vi "Phantom v7.3 lightweight controller.vi"() -> ()   [LabVIEW 2014]
uses:
  Program Files (x86)/National Instruments/LabVIEW 2011/instr.lib/Vision Research Phantom Series Labview Driver/_Type Defs/PHCon ACQUIPARAMS.ctl
  Program Files (x86)/National Instruments/LabVIEW 2011/instr.lib/Vision Research Phantom Series Labview Driver/_Type Defs/PhCon SyncImaging.ctl
  Program Files (x86)/National Instruments/LabVIEW 2011/instr.lib/Vision Research Phantom Series Labview Driver/_Type Defs/Rect.ctl
  Program Files (x86)/National Instruments/LabVIEW 2011/instr.lib/Vision Research Phantom Series Labview Driver/_Type Defs/PHCon Time64.ctl
  Program Files (x86)/National Instruments/LabVIEW 2011/instr.lib/Vision Research Phantom Series Labview Driver/_Type Defs/PhInt CFA.ctl
  Program Files (x86)/National Instruments/LabVIEW 2011/instr.lib/Vision Research Phantom Series Labview Driver/_Type Defs/enum buttons.ctl
  Program Files (x86)/National Instruments/LabVIEW 2011/instr.lib/Vision Research Phantom Series Labview Driver/_Type Defs/Point.ctl
  Program Files (x86)/National Instruments/LabVIEW 2011/instr.lib/Vision Research Phantom Series Labview Driver/_Type Defs/StampTime.ctl
  Program Files (x86)/National Instruments/LabVIEW 2011/instr.lib/Vision Research Phantom Series Labview Driver/_Type Defs/PHCon CINESTATUS.ctl
  Program Files (x86)/National Instruments/LabVIEW 2011/instr.lib/Vision Research Phantom Series Labview Driver/_Type Defs/PhCon Predefined Cines.ctl
  Program Files (x86)/National Instruments/LabVIEW 2011/instr.lib/Vision Research Phantom Series Labview Driver/_Type Defs/PHCon IMRANGE.ctl
  Program Files (x86)/National Instruments/LabVIEW 2011/instr.lib/Vision Research Phantom Series Labview Driver/_Type Defs/PhFile InfName.ctl
  Program Files (x86)/National Instruments/LabVIEW 2011/instr.lib/Vision Research Phantom Series Labview Driver/_Type Defs/PhInt PhProcessImage Selectors.ctl
panel:
  in  "Use timer":bool=TRUE
  out "Datarun timed out":bool
  in  "Save interval (shots)":u32
  out "Data run info":T1
  out "Run datasocket error":errorcluster
  in  "Zoom Factor":sgl(slide)=1.0 scale=0.0..10.0
  in  "Start recording":bool
  out "Last recording time":timestamp
  in  "Seconds between recordings":dbl format="%#_13g"
  out "Save path":path
  in  "Take picture":bool
  out "state":T2(ring)
  in  "Black Ref":bool
  in  "Recording":bool caption="Record?"
  out "Cine 1 Status":T3
  in  "Number of shots":i32
  in  "Frames After \nTrigger":i32
  in  "Frames Before \nTrigger":i32
  in  "Save StampTime":T4
  out "Save Progress":u8(slide) max=100 scale=0.0..100.0
  out "Error":errorcluster
  in  "error in":errorcluster
  out "Continue":bool
  in  "EXIT":bool
  in  "Trigger":bool
  in  "Update":bool
  in  "Parameters":T5
  out "Preview":picture
  out "CAR":T6[](array[typedef])
  in  "Current State":T7
  out "Serial":u32
  out "Camera Name":string
  out "Parameters":T8 {"CFA"."CFA" items=["CFA_NONE", "CFA_VRI", "CFA_VRIV6", "CFA_BAYER", "CFA_BAYERFLIP"]; "TriggerTime"."fractions" format="%32.0f"}
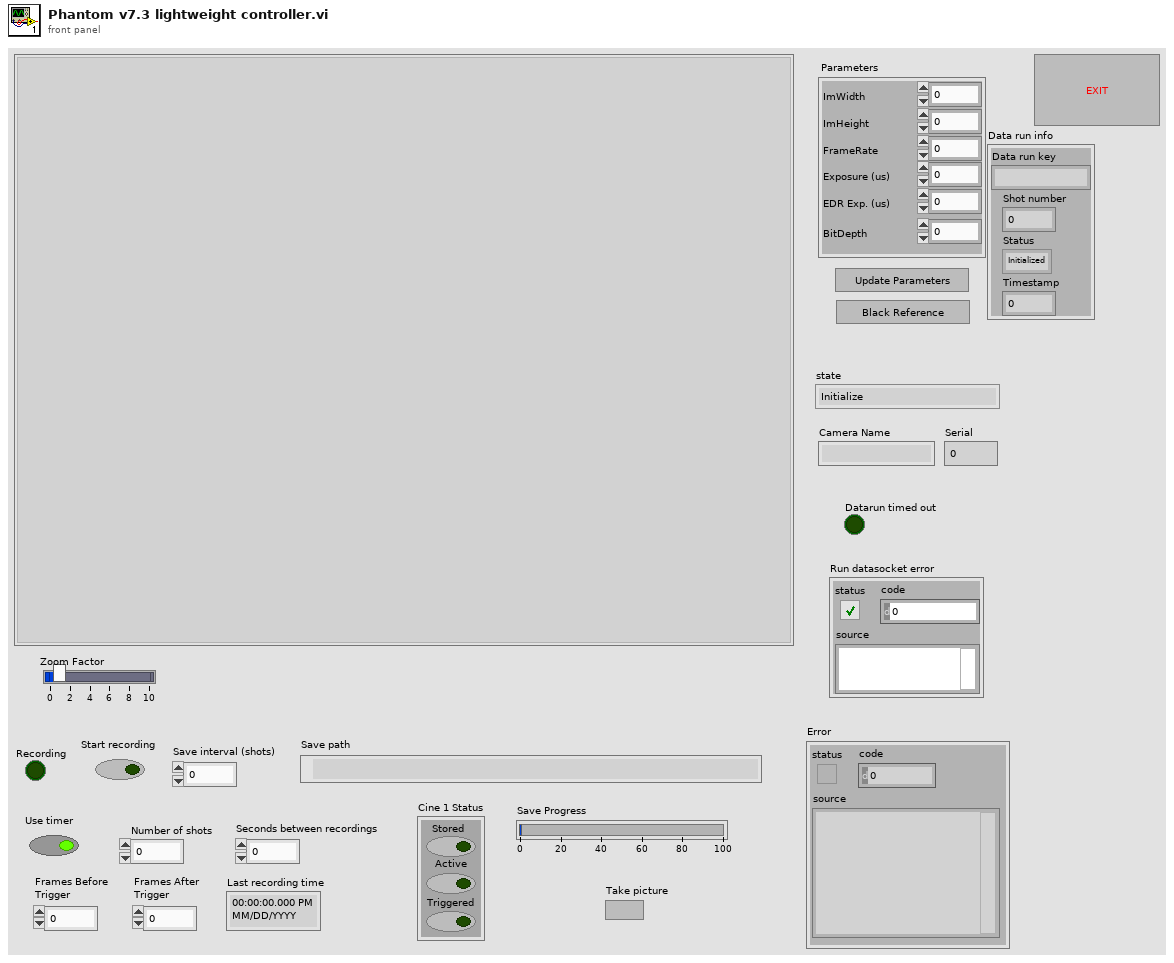
[diagram p1: front panel]
types:
  T1 = cluster{"Data run key":string, "Shot number":u32, "Status":enum16{"Initialized", "Running", "Aborted", "Default"}, "Timestamp":dbl}
  T2 = enum16{"Initialize", "Wait for Action", "Update", "Black Ref", "CTS", "Review", "End"}
  T3 = typedef "PHCon CINESTATUS.ctl" = cluster{"Stored":bool, "Active":bool, "Triggered":bool}
  T4 = typedef "StampTime.ctl" = enum32{"NoTimeStamp", "Time stamp", "", "Time stamp from trigger"}
  T5 = cluster{"ImWidth":u32, "ImHeight":u32, "FrameRate":u32, "Exposure (us)":u32, "EDR Exp. (us)":u32, "BitDepth":u32}
  T6 = typedef "Point.ctl" = cluster{"X":i32, "Y":i32}
  T7 = typedef "enum buttons.ctl" = enum16{"Initialize", "Wait for Action", "Update", "Capture", "Trigger", "Open Cine", "Save Cine", "CTS", "End"}
  T8 = typedef "PHCon ACQUIPARAMS.ctl" = cluster{"ImWidth":u32, "ImHeight":u32, "FrameRate":u32, "Exposure":u32, "EDRExposure":u32, "ImDelay":u32, "PTFrames":u32, "ImCount":u32, "SyncImaging":T9, "AutoExposure":u32, "AutoExpLevel":u32, "AutoExpSpeed":u32, "AutoExpRect":T10, "Recorded":bool, "TriggerTime":T11, "RecordedCount":u32, "FirstIm":i32, "FRPSteps":u32, "FRPImgNr":i32[], "FRPRate":u32[], "FRPExp":u32[], "Decimation":u32, "BitDepth":u32, "CamGainRed":u32, "CamGainGreen":u32, "CamGainBlue":u32, "CamGain":u32, "ShutterOff":bool, "CFA":T12, "CineName[256]":u8[], "Description[4096]":u8[], "FRPShape [16]":u32[]}
  T9 = typedef "PhCon SyncImaging.ctl" = enum32{"SYNC_INTERNAL", "SYNC_EXTERNAL", "SYNC_LOCKTOIRIG"}
  T10 = typedef "Rect.ctl" = cluster{"X":i32, "Y":i32, "Width":i32, "Height":i32}
  T11 = typedef "PHCon Time64.ctl" = cluster{"fractions":u32, "seconds":u32}
  T12 = typedef "PhInt CFA.ctl" = cluster{"CFA":u32, "VRIV6 Mask":cluster{"TL_GRAY":bool, "TR_GRAY":bool, "BL_GRAY":bool, "BR_GRAY":bool}}
  T13 = enum16{"Initialized", "Running", "Aborted", "Default"}
  T14 = cluster{"ImWidth":u32, "ImHeight":u32, "FrameRate":u32, "Exposure (us)":u32, "EDR Exp. (us)":u32, "ImDelay":u32, "Post Trig. Frames":u32, "ImCount":u32, "BitDepth":u32}
  T15 = typedef "PhCon Predefined Cines.ctl" = i32
  T16 = cluster{"pCS[0]":T3, "pCS[1]":T3, "pCS[2]":T3, "pCS[3]":T3, "pCS[4]":T3, "pCS[5]":T3, "pCS[6]":T3, "pCS[7]":T3, "pCS[8]":T3}
  T17 = typedef "PhInt PhProcessImage Selectors.ctl" = u16
  T18 = typedef "PhFile InfName.ctl" = u32
  T19 = typedef "PHCon IMRANGE.ctl" = cluster{"First":i32, "Cnt":u32}
  T20 = typedef "BITMAPINFO.ctl" = cluster{"BITMAPINFOHEADER":T21, "RGB Map":T22[]}
  T21 = typedef "BITMAPINFOHEADER.ctl" = cluster{"biSize":u32, "biWidth":i32, "biHeight":i32, "biPlanes":u16, "biBitCount":u16, "biCompression":u32, "biSizeImage":u32, "biXPelsPerMeter":i32, "biYPelsPerMeter":i32, "biClrUsed":u32, "biClrImportant":u32}
  T22 = typedef "RGBQUAD.ctl" = cluster{"rgbBlue":u8, "rgbGreen":u8, "rgbRed":u8, "rgbResevered":u8}
  T23 = typedef "PhInt IH.ctl" = cluster{"biSize":u32, "biWidth":i32, "biHeight":i32, "biPlanes":u16, "biBitCount":u16, "biCompresssion":u32, "biSizeImage":u32, "biXPelsPerMeter":i32, "biYPelsPerMeter":i32, "biClrUsed":u32, "biClrImportant":u32, "BlackLevel":i32, "WhiteLevel":i32}
  T24 = typedef "PHCon CAMERAOPTIONS.ctl" = cluster{"OSD":u32, "VideoSystem":T25, "ModulatedIRIG":bool, "RisingEdge":bool, "FilterTime":u32, "MemGate":bool, "StartInRec":bool, "Color":bool, "TestImage":bool, "OSDColor [8]":T22[], "OSDOpaque":bool, "OSDLeft":i32, "OSDTop":i32, "OSDBottom":i32, "ImageX":i32, "ImageY":i32, "AutoSaveNVM":bool, "AutoSaveFile":bool, "AutoPlay":bool, "AutoCapture":bool, "Filename":u8[], "SaveRng":T19, "LongReady":bool, "RealTimeOutput":bool, "RangeData":u32, "SourceCamSer":u32, "SliceNr":u32, "SliceCnt":u32, "FRPi3Trig":bool, "UT":u32, "AutoSaveFormat":i8, "SourceCamVer":u32, "RAMBitDepth":u32, "VideoTone":i32, "VideoZoom":i32, "FormatWidth":i32, "FormatHeight":i32, "AutoPlayCnt":u32, "OSDDisable":u32, "RecToMag":bool, "IrigOut":bool, "FormatXOffset":i32, "FormatYOffset":i32}
  T25 = typedef "PhCon VideoSystem.ctl" = u32
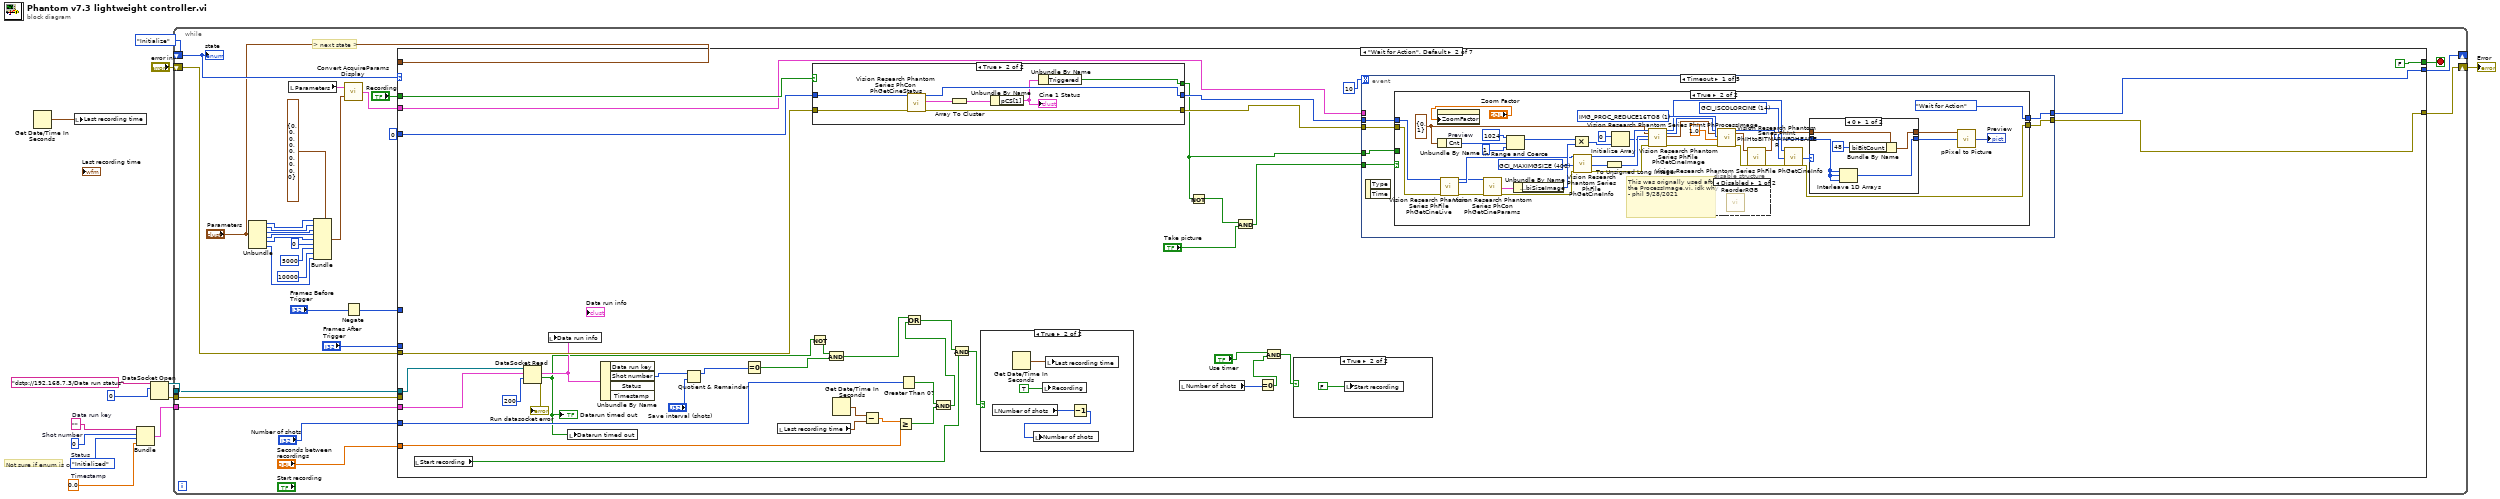
[diagram p0: block diagram]
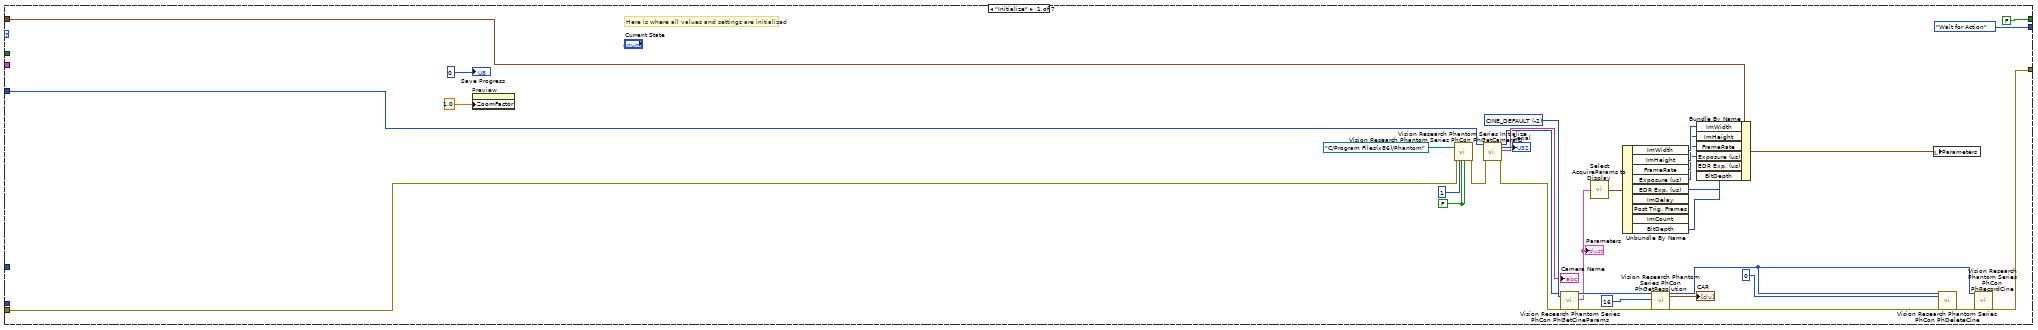
[diagram p2: hidden frame]
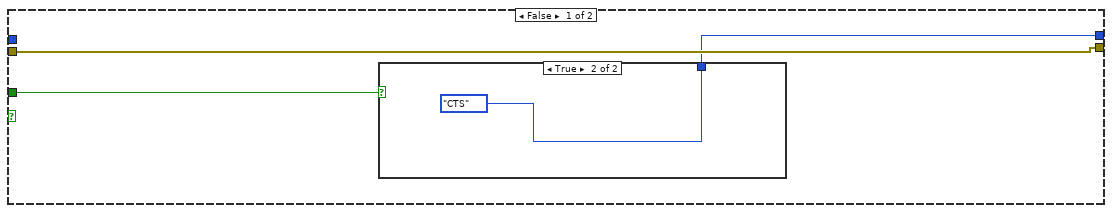
[diagram p5: hidden frame]
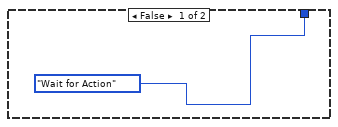
[diagram p6: hidden frame]
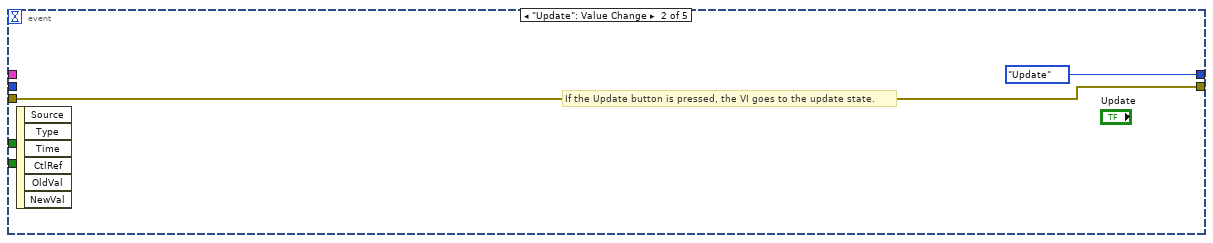
[diagram p9: hidden frame]
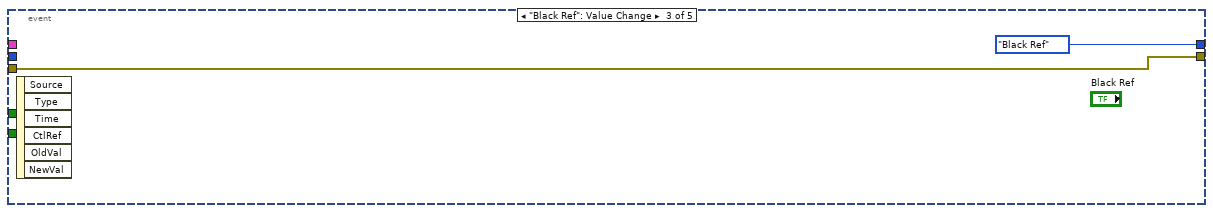
[diagram p10: hidden frame]
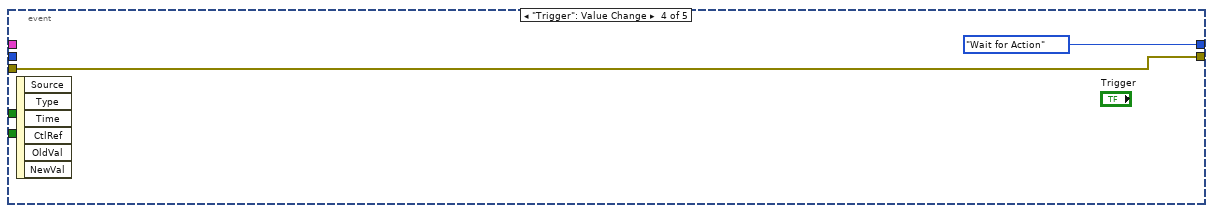
[diagram p11: hidden frame]
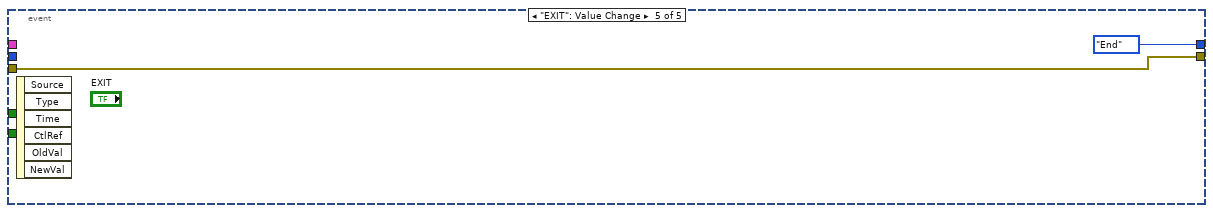
[diagram p12: hidden frame]
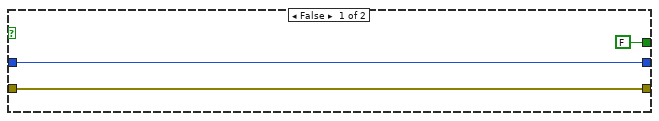
[diagram p13: hidden frame]
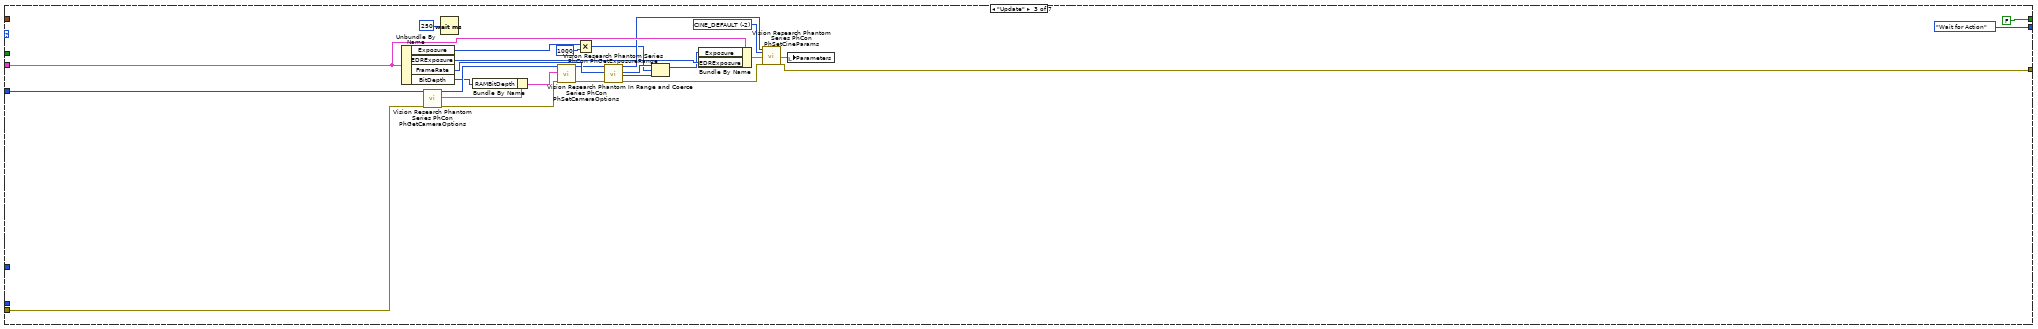
[diagram p14: hidden frame]
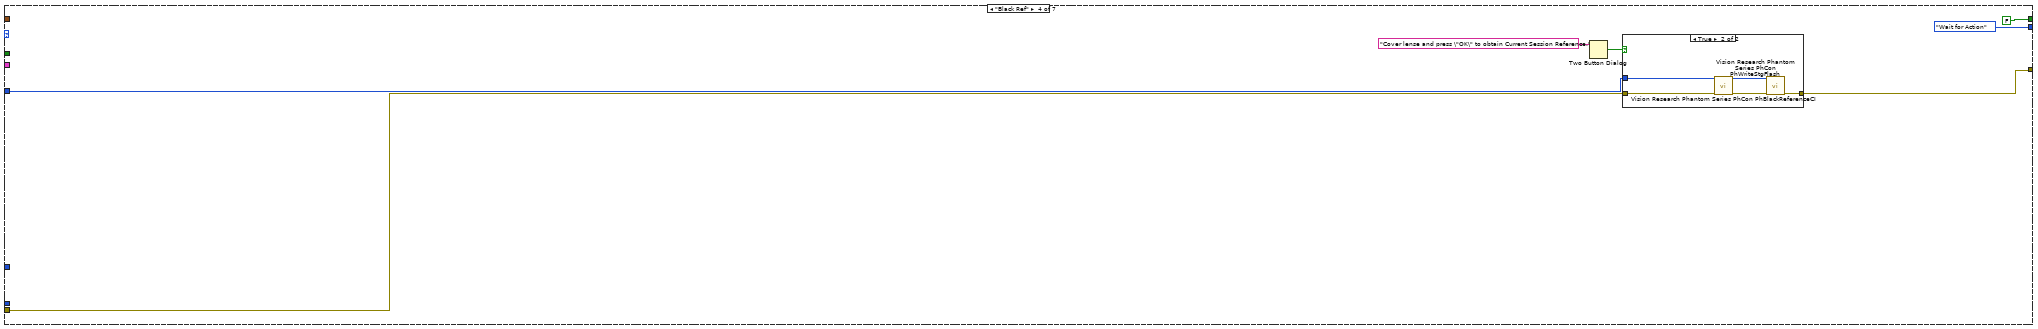
[diagram p15: hidden frame]
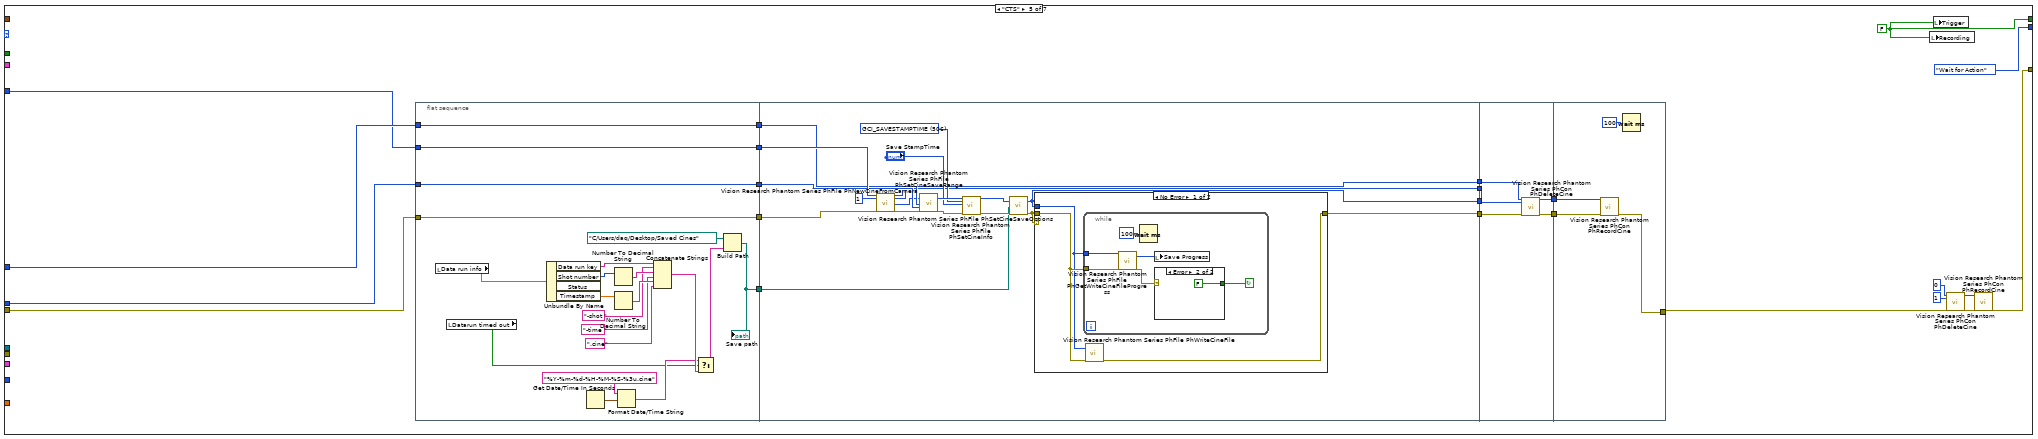
[diagram p17: hidden frame]
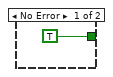
[diagram p18: hidden frame]
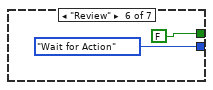
[diagram p20: hidden frame]
diagram:
  w8 = 0.0  # Timestamp
  w7 = T13."Initialized"  # Status
  w6 = u32 0  # Shot number
  w5 = ""  # Data run key
  # "Not sure if enum is correct"
  n1 = Get Date/Time In Seconds() -> (seconds since 1Jan1904=w1:timestamp)
  n2 = local write "Last recording time"(w1) -> ()
  n3 = Bundle("Data run key"=w5, "Shot number"=w6, "Status"=w7, "Timestamp"=w8) -> (w4:T1)  [unwired: 1 in]
  n4 = DataSocket Open(10:0, 11:"dstp://192.168.7.3/Data run status") -> (0:w2:errorcluster, 3:w3:refnum<k13>)  [unwired: 2 in]
  n5 = while {
    shift-right: [w42] -> _
    shift-left: T2."Initialize" -> [w41]
    shift-right: [w39] -> w13
    shift-left: "error in" -> [w31]
    tunnel: w3 -> [w18]
    tunnel: w4 -> [w17]
    tunnel: w2 -> [w16]
    stop <- w40 stop-if-true
    # "> next state >"
    n6 = Unbundle("Parameters") -> ("ImWidth"=w30:u32, "ImHeight"=w29:u32, "FrameRate"=w28:u32, "Exposure (us)"=w27:u32, "EDR Exp. (us)"=w26:u32, "BitDepth"=w21:u32)
    n7 = local read "Parameters"() -> (w37:T8)
    n8 = Bundle(cluster=T14 {"ImWidth"=0, "ImHeight"=0, "FrameRate"=0, "Exposure (us)"=0, "EDR Exp. (us)"=0, "ImDelay"=0, "Post Trig. Frames"=0, "ImCount"=0, "BitDepth"=0} ("ACQUIPARAMS Display"), "ImWidth"=w30, "ImHeight"=w29, "FrameRate"=w28, "Exposure (us)"=w27, "EDR Exp. (us)"=w26, "ImDelay"=u32 0 ("x"), "Post Trig. Frames"=u32 5000 ("x"), "ImCount"=u32 10000 ("x"), "BitDepth"=w21) -> (w22:T14)
    n9 = call "Convert AcquireParams Display.vi"("ACQUIPARAMS Display"=w22, "ACQUIPARAMS [in]"=w37) -> ("ACQUIPARAMS [out]"=w38:T8)
    n10 = Negate(x="Frames Before \nTrigger") -> (-x=w32:i32)
    n11 = case shown="\"Wait for Action\", Default" w41 {
      selector: w41 -> [_ _ _ _ _ _ w331]
      tunnel: w38 -> [_ w109 w223 _ _ _ _]
      tunnel: [T2."Wait for Action" w105 T2."Wait for Action" T2."Wait for Action" T2."Wait for Action" T2."Wait for Action" w331] -> w42
      tunnel: [FALSE FALSE FALSE FALSE w256 FALSE TRUE] -> w40
      tunnel: w31 -> [w61 w117 w208 w230 w249 _ w329]
      tunnel: [w58 w106 w221 w229 w262 _ w327] -> w39
      tunnel: u32 0 ("Camera Number") -> [w66 w116 w207 w231 w246 _ _]
      tunnel: "Frames After \nTrigger" -> [_ _ _ _ w247 _ _]
      tunnel: w32 -> [_ _ _ _ w248 _ _]
      tunnel: "Recording" -> [_ w115 _ _ _ _ _]
      tunnel: "Parameters" -> [w44 _ _ _ _ _ _]
      tunnel: w18 -> [_ w93 _ _ _ _ _]
      tunnel: w17 -> [_ w92 _ _ _ _ _]
      tunnel: w16 -> [_ _ _ _ _ _ _]
      tunnel: "Number of shots" -> [_ w103 _ _ _ _ _]
      tunnel: "Seconds between recordings" -> [_ w99 _ _ _ _ _]
      frame "Initialize" {
        w69 = FALSE ("ID Query (T: Check)")
        w72 = T15 -2 items=["CINE_DEFAULT "=-2, "CINE_CURRENT "=-1, "CINE_PREVIEW  "=0, "CINE_FIRST    "=1] ("Cine")
        # "Here is where all values and settings are initialized"
        n12 = property on="Preview" class="Pict"("ZoomFactor"=sgl 1.0 ("Zoom Factor")) -> ()  [unwired: 2 in, 2 out]
        n13 = call "Vision Research Phantom Series Initialize.vi"("Storage Path (\"\")"=path "C:/Program Files(x86)/Phantom" ("Storage Path (\"\")"), "error in (no error)"=w61, "CallID"=u32 1, "ID Query (T: Check)"=w69, "Reset (F: Don't Reset)"=w69) -> ("Error Out"=w68:errorcluster)  [unwired: 14 out]
        n14 = call "Vision Research Phantom Series PhCon PhGetCameraID.vi"("CN in"=w66, "Error In (no error)"=w68) -> ("CN out"=w59:u32, "pSerial"=→"Serial":u32, "pCameraName"=→"Camera Name":string, "Error Out"=w60:errorcluster)  [unwired: 1 in, 13 out]
        n15 = call "Vision Research Phantom Series PhCon PhGetCineParams.vi"("CN in"=w59, "Cine"=w72, "Error In (no error)"=w60) -> ("CN out"=w75:u32, "ACQUIPARAMS"=w64:T8, "Error Out"=w65:errorcluster)  [unwired: 1 in, 13 out]
        "Parameters" <- w64
        n16 = call "Select AcquireParams to Display.vi"("ACQUIPARAMS"=w64) -> ("ACQUIPARAMS Display"=w51:T14)
        n17 = Unbundle By Name(w51) -> ("ImWidth"=w50:u32, "ImHeight"=w49:u32, "FrameRate"=w48:u32, "Exposure (us)"=w47:u32, "EDR Exp. (us)"=w45:u32, "BitDepth"=w46:u32)  [unwired: 3 out]
        n18 = call "Vision Research Phantom Series PhCon PhGetResolution.vi"("CN in"=w75, "pCnt"=16, "Error In (no error)"=w65) -> ("CN out"=w56:u32, "CAR"=→"CAR":T6[], "Error Out"=w55:errorcluster)  [unwired: 2 in, 12 out]
        n19 = Bundle By Name(cluster=w44, "ImWidth"=w50, "ImHeight"=w49, "FrameRate"=w48, "Exposure (us)"=w47, "EDR Exp. (us)"=w45, "BitDepth"=w46) -> (w43:T5)
        n20 = local write "Parameters"(w43) -> ()
        n21 = call "Vision Research Phantom Series PhCon PhDeleteCine.vi"("CN in"=w56, "Cine"=0, "Error In (no error)"=w55) -> ("Error Out"=w54:errorcluster)  [unwired: 15 in, 1 out]
        n22 = call "Vision Research Phantom Series PhCon PhRecordCine.vi"("CN in"=w56, "Error In (no error)"=w54) -> ("Error Out"=w58:errorcluster)  [unwired: 1 in, 16 out]
        "Save Progress" <- u8 0 ("Value")
      }
      frame "Wait for Action", Default {
        n23 = local read "Start recording"() -> (w81:bool)
        n24 = DataSocket Read(9:200, 10:w92, 11:w93) -> (0:→"Run datasocket error":errorcluster, 1:w86:bool, 2:w91:T1)  [unwired: 2 in, 4 out]
        "Datarun timed out" <- w86
        n25 = local write "Data run info"(w91) -> ()
        n26 = local write "Datarun timed out"(w86) -> ()
        n27 = Unbundle By Name(w91) -> ("Shot number"=w90:u32)  [unwired: 3 out]
        n28 = Quotient & Remainder(x=w90, y="Save interval (shots)") -> (x-y*floor(x/y)=w88:u32)  [unwired: 1 out]
        n29 = Equal To 0?(x=w88) -> (x = 0?=w87:bool)
        n30 = local read "Last recording time"() -> (w101:timestamp)
        n31 = Not(x=w86) -> (.not. x?=w85:bool)
        n32 = case shown="True" w115 {
          tunnel: w117 -> [w191 w199]
          tunnel: w116 -> [w190 w198]
          tunnel: [w190 w197] -> w108
          tunnel: [FALSE ("Triggered") w193] -> w104
          tunnel: [w191 w192] -> w107
          frame False {
          }
          frame True {
            n33 = call "Vision Research Phantom Series PhCon PhGetCineStatus.vi"("CN in"=w198, "Error In (no error)"=w199) -> ("CN out"=w197:u32, "pCS"=w196:T3[], "Error Out"=w192:errorcluster)  [unwired: 15 in]
            n34 = Array To Cluster(array=w196) -> (cluster=w195:T16)
            n35 = Unbundle By Name(w195) -> ("pCS[1]"=w194:T3)
            "Cine 1 Status" <- w194
            n36 = Unbundle By Name(w194) -> ("Triggered"=w193:bool)
          }
        }
        n37 = And(x=w85, y=w87) -> (x .and. y?=w84:bool)
        n38 = Get Date/Time In Seconds() -> (seconds since 1Jan1904=w102:timestamp)
        n39 = Subtract(x=w102, y=w101) -> (x-y=w100:dbl)
        n40 = Greater Or Equal?(x=w100, y=w99) -> (x >= y?=w97:bool)
        n41 = Greater Than 0?(x=w103) -> (x > 0?=w98:bool)
        n42 = And(x=w98, y=w97) -> (x .and. y?=w83:bool)
        n43 = Or(x=w84, y=w83) -> (x .or. y?=w82:bool)
        n44 = And(x=w82, y=w81) -> (x .and. y?=w80:bool)
        n45 = case shown="True" w80 {
          frame False {
          }
          frame True {
            n46 = local read "Number of shots"() -> (w121:i32)
            n47 = Get Date/Time In Seconds() -> (seconds since 1Jan1904=w120:timestamp)
            n48 = local write "Recording"(TRUE ("Record?")) -> ()
            n49 = local write "Last recording time"(w120) -> ()
            n50 = Decrement(x=w121) -> (x-1=w119:i32)
            n51 = local write "Number of shots"(w119) -> ()
          }
        }
        n52 = local read "Number of shots"() -> (w96:i32)
        n53 = Not(x=w104) -> (.not. x?=w112:bool)
        n54 = And(x=w112, y="Take picture") -> (x .and. y?=w110:bool)
        n55 = Equal To 0?(x=w96) -> (x = 0?=w78:bool)
        n56 = And(x="Use timer", y=w78) -> (x .and. y?=w77:bool)
        n57 = case shown="True" w77 {
          frame False {
          }
          frame True {
            n58 = local write "Start recording"(FALSE ("Start recording")) -> ()
          }
        }
        n59 = event shown="[0] Timeout" {
          selector: _ -> [_ _ _ _ _]
          dyn-events: _ -> [_ _ _ _ _]
          timeout: 10 -> [_ _ _ _ _]
          tunnel: [w125 T2."Update" T2."Black Ref" T2."Wait for Action" T2."End"] -> w105
          tunnel: w107 -> [w127 w182 w183 w186 w188]
          tunnel: [w128 w182 w183 w186 w188] -> w106
          tunnel: w109 -> [_ _ _ _ _]
          tunnel: w108 -> [w126 _ _ _ _]
          tunnel: w110 -> [w124 _ _ _ _]
          tunnel: w104 -> [w123 _ _ _ _]
          event Timeout {
            n60 = event-data() -> ()  [unwired: 3 out]
            n61 = case shown="True" w124 {
              tunnel: [w131 w153] -> w128
              tunnel: w127 -> [w131 w149]
              tunnel: w126 -> [_ w148]
              tunnel: [w129 T2."Wait for Action"] -> w125
              tunnel: w123 -> [w130 _]
              frame False {
                n62 = case shown="True" w130 {
                  tunnel: [T2."Wait for Action" T2."CTS"] -> w129
                  frame False {
                  }
                  frame True {
                  }
                }
              }
              frame True {
                w155 = T17 1 items=["IMG_PROC_REDUCE16TO8"=1] ("procID")
                w158 = T18 14 items=["GCI_CFA"=0, "GCI_FRAMERATE"=1, "GCI_EXPOSURE"=2, "GCI_AUTOEXPOSURE"=3, "GCI_REALBPP"=4, "GCI_CAMERASERIAL"=5, "GCI_HEADSERIAL0"=6, "GCI_HEADSERIAL1"=7, "GCI_HEADSERIAL2"=8, "GCI_HEADSERIAL3"=9, "GCI_TRIGTIMESEC"=10, "GCI_TRIGTIMEFR"=11, "GCI_ISFILECINE"=12, "GCI_IS16BPPCINE"=13, "GCI_ISCOLORCINE"=14, "GCI_ISMULTIHEADCINE"=15, "GCI_EXPOSURENS"=16, "GCI_EDREXPOSURENS"=17, "GCI_FRAMEDELAYNS"=19, "GCI_FROMFILETYPE"=20, "GCI_COMPRESSION"=21, "GCI_CAMERAVERSION"=22, "GCI_ROTATE"=23, "GCI_IMWIDTH"=24, "GCI_IMHEIGHT"=25, "GCI_IMWIDTHACQ"=26, "GCI_IMHEIGHTACQ"=27, "GCI_POSTTRIGGER"=28, "GCI_IMAGECOUNT"=29, "GCI_TOTALIMAGECOUNT"=30, "GCI_TRIGFRAME"=31, "GCI_AUTOEXPLEVEL"=32, "GCI_AUTOEXPTOP"=33, "GCI_AUTOEXPLEFT"=34, "GCI_AUTOEXPBOTTOM"=35, "GCI_AUTOEXPRIGHT"=36, "GCI_RECORDINGTIMEZONE"=37, "GCI_FIRSTIMAGENO"=38, "GCI_FIRSTMOVIEIMAGE"=39, "GCI_CINENAME"=40, "GCI_FRPSTEPS"=100, "GCI_FRP1X"=101, "GCI_FRP1Y"=102, "GCI_FRP2X"=103, "GCI_FRP2Y"=104, "GCI_FRP3X"=105, "GCI_FRP3Y"=106, "GCI_FRP4X"=107, "GCI_FRP4Y"=108, "GCI_WRITEERR"=109, "GCI_LENSDESCRIPTION"=110, "GCI_LENSAPERATURE"=111, "GCI_LENSFOCALLENGTH"=112, "GCI_WB"=200, "GCI_WBVIEW"=201, "GCI_BRIGHT"=202, "GCI_CONTRAST"=203, "GCI_GAMMA"=204, "GCI_GAMMAR"=223, "GCI_GAMMAB"=224, "GCI_SATURATION"=205, "GCI_HUE"=206, "GCI_FLIPH"=207, "GCI_FLIPV"=208, "GCI_FILTERCODE"=209, "GCI_IMFILTER"=210, "GCI_INTALGO"=211, "GCI_PEDESTALR"=212, "GCI_PEDESTALG"=213, "GCI_PEDESTALB"=214, "GCI_FLARE"=225, "GCI_CHROMA"=226, "GCI_TONE"=227, "GCI_ENABLEMATRICES"=228, "GCI_USERMATRIX"=229, "GCI_RESAMPLEACTIVE"=215, "GCI_RESAMPLEWIDTH"=216, "GCI_RESAMPLEHEIGHT"=217, "GCI_CROPACTIVE"=218, "GCI_CROPRECTANGLE"=219, "GCI_OFFSET16_8"=220, "GCI_GAIN16_8"=221, "GCI_DEMOSAICINGFUNCPTR"=222, "GCI_VFLIPVIEWACTIVE"=300, "GCI_MAXIMGSIZE"=400, "GCI_FRPIMGNOARRAY"=450, "GCI_FRPRATEARRAY"=451, "GCI_FRPSHAPEARRAY"=452, "GCI_TRIGTC"=470, "GCI_TRIGTCU"=471, "GCI_PBRATE"=472, "GCI_TCRATE"=473, "GCI_SAVERANGE"=500, "GCI_SAVEFILENAME"=501, "GCI_SAVEFILETYPE"=502, "GCI_SAVE16BIT"=503, "GCI_SAVEPACKED"=504, "GCI_SAVEXML"=505, "GCI_SAVESTAMPTIME"=506, "GCI_SAVEAVIFRAMERATE"=520, "GCI_SAVEAVICOMPRESSORLIST"=521, "GCI_SAVEAVICOMPRESSORINDEX"=522, "GCI_SAVEDPXLSB"=530, "GCI_SAVEDPXTO10BPS"=531, "GCI_SAVEDPXDATAPACKING"=532, "GCI_SAVEDPX10BITLOG"=533, "GCI_SAVEDPXEXPORTLOGLUT"=534, "GCI_SAVEDPX10BITLOGREFWHITE"=535, "GCI_SAVEDPX10BITLOGREFBLACK"=536, "GCI_SAVEDPX10BITLOGGAMMA"=537, "GCI_SAVEDPX10BITLOGFILMGAMMA"=538, "GCI_SAVEQTPLAYBACKRATE"=550, "GCI_SAVECCIQUALITY"=560, "GCI_UNCALIBRATEDIMAGE"=600, "GCI_NOPROCESSING"=601, "GCI_BADPIXELREPAIR"=602] ("InfName")
                w173 = T18 400 items=["GCI_CFA"=0, "GCI_FRAMERATE"=1, "GCI_EXPOSURE"=2, "GCI_AUTOEXPOSURE"=3, "GCI_REALBPP"=4, "GCI_CAMERASERIAL"=5, "GCI_HEADSERIAL0"=6, "GCI_HEADSERIAL1"=7, "GCI_HEADSERIAL2"=8, "GCI_HEADSERIAL3"=9, "GCI_TRIGTIMESEC"=10, "GCI_TRIGTIMEFR"=11, "GCI_ISFILECINE"=12, "GCI_IS16BPPCINE"=13, "GCI_ISCOLORCINE"=14, "GCI_ISMULTIHEADCINE"=15, "GCI_EXPOSURENS"=16, "GCI_EDREXPOSURENS"=17, "GCI_FRAMEDELAYNS"=19, "GCI_FROMFILETYPE"=20, "GCI_COMPRESSION"=21, "GCI_CAMERAVERSION"=22, "GCI_ROTATE"=23, "GCI_IMWIDTH"=24, "GCI_IMHEIGHT"=25, "GCI_IMWIDTHACQ"=26, "GCI_IMHEIGHTACQ"=27, "GCI_POSTTRIGGER"=28, "GCI_IMAGECOUNT"=29, "GCI_TOTALIMAGECOUNT"=30, "GCI_TRIGFRAME"=31, "GCI_AUTOEXPLEVEL"=32, "GCI_AUTOEXPTOP"=33, "GCI_AUTOEXPLEFT"=34, "GCI_AUTOEXPBOTTOM"=35, "GCI_AUTOEXPRIGHT"=36, "GCI_RECORDINGTIMEZONE"=37, "GCI_FIRSTIMAGENO"=38, "GCI_FIRSTMOVIEIMAGE"=39, "GCI_CINENAME"=40, "GCI_FRPSTEPS"=100, "GCI_FRP1X"=101, "GCI_FRP1Y"=102, "GCI_FRP2X"=103, "GCI_FRP2Y"=104, "GCI_FRP3X"=105, "GCI_FRP3Y"=106, "GCI_FRP4X"=107, "GCI_FRP4Y"=108, "GCI_WRITEERR"=109, "GCI_LENSDESCRIPTION"=110, "GCI_LENSAPERATURE"=111, "GCI_LENSFOCALLENGTH"=112, "GCI_WB"=200, "GCI_WBVIEW"=201, "GCI_BRIGHT"=202, "GCI_CONTRAST"=203, "GCI_GAMMA"=204, "GCI_GAMMAR"=223, "GCI_GAMMAB"=224, "GCI_SATURATION"=205, "GCI_HUE"=206, "GCI_FLIPH"=207, "GCI_FLIPV"=208, "GCI_FILTERCODE"=209, "GCI_IMFILTER"=210, "GCI_INTALGO"=211, "GCI_PEDESTALR"=212, "GCI_PEDESTALG"=213, "GCI_PEDESTALB"=214, "GCI_FLARE"=225, "GCI_CHROMA"=226, "GCI_TONE"=227, "GCI_ENABLEMATRICES"=228, "GCI_USERMATRIX"=229, "GCI_RESAMPLEACTIVE"=215, "GCI_RESAMPLEWIDTH"=216, "GCI_RESAMPLEHEIGHT"=217, "GCI_CROPACTIVE"=218, "GCI_CROPRECTANGLE"=219, "GCI_OFFSET16_8"=220, "GCI_GAIN16_8"=221, "GCI_DEMOSAICINGFUNCPTR"=222, "GCI_VFLIPVIEWACTIVE"=300, "GCI_MAXIMGSIZE"=400, "GCI_FRPIMGNOARRAY"=450, "GCI_FRPRATEARRAY"=451, "GCI_FRPSHAPEARRAY"=452, "GCI_TRIGTC"=470, "GCI_TRIGTCU"=471, "GCI_PBRATE"=472, "GCI_TCRATE"=473, "GCI_SAVERANGE"=500, "GCI_SAVEFILENAME"=501, "GCI_SAVEFILETYPE"=502, "GCI_SAVE16BIT"=503, "GCI_SAVEPACKED"=504, "GCI_SAVEXML"=505, "GCI_SAVESTAMPTIME"=506, "GCI_SAVEAVIFRAMERATE"=520, "GCI_SAVEAVICOMPRESSORLIST"=521, "GCI_SAVEAVICOMPRESSORINDEX"=522, "GCI_SAVEDPXLSB"=530, "GCI_SAVEDPXTO10BPS"=531, "GCI_SAVEDPXDATAPACKING"=532, "GCI_SAVEDPX10BITLOG"=533, "GCI_SAVEDPXEXPORTLOGLUT"=534, "GCI_SAVEDPX10BITLOGREFWHITE"=535, "GCI_SAVEDPX10BITLOGREFBLACK"=536, "GCI_SAVEDPX10BITLOGGAMMA"=537, "GCI_SAVEDPX10BITLOGFILMGAMMA"=538, "GCI_SAVEQTPLAYBACKRATE"=550, "GCI_SAVECCIQUALITY"=560, "GCI_UNCALIBRATEDIMAGE"=600, "GCI_NOPROCESSING"=601, "GCI_BADPIXELREPAIR"=602] ("InfName")
                w145 = T19 {"First"=0, "Cnt"=1} ("pRng")
                # "This was orignally used after the ProcessImage.vi. idk why\n- phil 9/28/2021"
                n63 = property on="Preview" class="Pict"("ZoomFactor"="Zoom Factor") -> ()  [unwired: 2 in, 2 out]
                n64 = Unbundle By Name(w145) -> ("Cnt"=w167:u32)
                n65 = call "Vision Research Phantom Series PhFile PhGetCineLive.vi"("CN (in)"=w148, "Error In (no error)"=w149) -> ("CN (out)"=w151:u32, "pCH (out)"=w152:u32, "Error Out"=w150:errorcluster)  [unwired: 1 in, 14 out]
                n66 = call "Vision Research Phantom Series PhCon PhGetCineParams.vi"("CN in"=w151, "Error In (no error)"=w150) -> ("pBMI"=w166:T20, "Error Out"=w165:errorcluster)  [unwired: 2 in, 14 out]
                n67 = In Range and Coerce(upper limit=u32 1024, x=w167, lower limit=u32 1) -> (coerced(x)=w168:u32)  [unwired: 1 out]
                n68 = Unbundle By Name(w166) -> ("BITMAPINFOHEADER.biSizeImage"=w171:u32)
                n69 = call "Vision Research Phantom Series PhFile PhGetCineInfo.vi"("CH in"=w152, "InfName"=w173, "Error In (no error)"=w165) -> ("CH out"=w146:u32, "pInfVal out"=w164:i32, "Error Out"=w142:errorcluster)  [unwired: 1 in, 13 out]
                n70 = Compound Arithmetic op=MULTIPLY(w168, w171) -> (w172:u32)
                n71 = To Unsigned Long Integer(number=w164) -> (unsigned 32bit integer=w144:u32)
                n72 = Initialize Array(u16 0 ("element"), w172) -> (w143:u16[])
                n73 = call "Vision Research Phantom Series PhFile PhGetCineImage.vi"("hC [in]"=w146, "pRng [in]"=w145, "bufferByteSize [in]"=w144, "pPixelBuffer [in]"=w143, "Error In (no error)"=w142) -> ("hC [out]"=w141:u32, "pPixelBuffer [out]"=w137:u16[], "IH [out]"=w140:T23, "Error Out"=w139:errorcluster)  [unwired: 11 in]
                n74 = disable-structure shown="Disabled" {
                  frame Disabled {
                    n75 = call "ReorderRGB.vi"() -> ()  [unwired: 1 in, 1 out]
                  }
                  frame Enabled {
                  }
                }
                n76 = call "Vision Research Phantom Series PhInt PhProcessImage.vi"("pPixelSrc [in]"=w137, "IH [in]"=w140, "procID"=w155, "pProcParams"=1.0, "Error In (no error)"=w139) -> ("pPixelDest [out]"=w134:u8[], "IH [out]"=w162:T23, "Error Out"=w161:errorcluster)  [unwired: 1 in, 11 out]
                n77 = call "Vision Research Phantom Series PhInt PhIHtoBITMAPINFOHEADER.vi"("IH"=w162, "Error In (no error)"=w161) -> ("BITMAPINFOHEADER"=w159:T21, "Error Out"=w154:errorcluster)  [unwired: 1 in, 15 out]
                n78 = call "Vision Research Phantom Series PhFile PhGetCineInfo.vi"("CH in"=w141, "InfName"=w158, "Error In (no error)"=w154) -> ("pInfVal out"=w160:i32, "Error Out"=w153:errorcluster)  [unwired: 1 in, 14 out]
                n79 = case shown="0" w160 {
                  tunnel: [w177 w180] -> w136
                  tunnel: w134 -> [w178 w180]
                  tunnel: w159 -> [w176 w179]
                  tunnel: [w175 w179] -> w157
                  frame 0 {
                    n80 = Interleave 1D Arrays(w178, w178, w178) -> (w177:u8[])
                    n81 = Bundle By Name(cluster=w176, "biBitCount"=u16 48) -> (w175:T21)
                  }
                  frame 1, Default {
                  }
                }
                n82 = call "pPixel to Picture.vi"("pPixel"=w136, "BITMAPINFOHEADER"=w157) -> ("Preview"=→"Preview":picture)  [unwired: 1 in]
              }
            }
          }
          event "Update": Value Change {
            # "If the Update button is pressed, the VI goes to the update state."
            n83 = event-data() -> ()  [unwired: 7 out]
          }
          event "Black Ref": Value Change {
            n84 = event-data() -> ()  [unwired: 7 out]
          }
          event "Trigger": Value Change {
            n85 = event-data() -> ()  [unwired: 7 out]
          }
          event "EXIT": Value Change {
            n86 = event-data() -> ()  [unwired: 7 out]
          }
        }
      }
      frame "Update" {
        w225 = T15 -2 items=["CINE_DEFAULT "=-2, "CINE_CURRENT "=-1, "CINE_PREVIEW  "=0, "CINE_FIRST    "=1] ("Cine")
        n87 = Unbundle By Name(w223) -> ("Exposure"=w212:u32, "EDRExposure"=w214:u32, "FrameRate"=w217:u32, "BitDepth"=w200:u32)
        n88 = call "Vision Research Phantom Series PhCon PhGetCameraOptions.vi"("CN in"=w207, "Error In (no error)"=w208) -> ("CN out"=w203:u32, "CAMERAOPTIONS"=w202:T24, "Error Out"=w204:errorcluster)  [unwired: 1 in, 14 out]
        n89 = Wait (ms)(milliseconds to wait=u32 250) -> ()  [unwired: 1 out]
        n90 = Bundle By Name(cluster=w202, "RAMBitDepth"=w200) -> (w201:T24)
        n91 = call "Vision Research Phantom Series PhCon PhSetCameraOptions.vi"("CN in"=w203, "CAMERAOPTIONS"=w201, "Error In (no error)"=w204) -> ("CN out"=w206:u32, "Error Out"=w205:errorcluster)  [unwired: 1 in, 14 out]
        n92 = Multiply(x=w212, y=u32 1000 ("x")) -> (x*y=w210:u32)
        n93 = call "Vision Research Phantom Series PhCon PhGetExposureRange.vi"("CN in"=w206, "FrameRate"=w217, "Error In (no error)"=w205) -> ("CN out"=w218:u32, "pMaxExposure"=w213:u32, "pMinExposure"=w215:u32, "Error Out"=w216:errorcluster)  [unwired: 1 in, 12 out]
        n94 = In Range and Coerce(upper limit=w213, x=w210, lower limit=w215) -> (coerced(x)=w209:u32)  [unwired: 1 out]
        n95 = Bundle By Name(cluster=w223, "Exposure"=w209, "EDRExposure"=w214) -> (w222:T8)
        n96 = call "Vision Research Phantom Series PhCon PhSetCineParams.vi"("CN in"=w218, "Cine"=w225, "ACQUIPARAMS"=w222, "Error In (no error)"=w216) -> ("ACQUIPARAMS out"=w220:T8, "Error Out"=w221:errorcluster)  [unwired: 1 in, 13 out]
        n97 = local write "Parameters"(w220) -> ()
      }
      frame "Black Ref" {
        n98 = Two Button Dialog(message="Cover lense and press \"OK\" to obtain Current Session Reference.") -> (T button?=w227:bool)  [unwired: 2 in]
        n99 = case shown="True" w227 {
          tunnel: w231 -> [_ w239]
          tunnel: w230 -> [w234 w238]
          tunnel: [w234 w236] -> w229
          frame False {
          }
          frame True {
            n100 = call "Vision Research Phantom Series PhCon PhBlackReferenceCI.vi"("CN in"=w239, "Error In (no error)"=w238) -> ("CN out"=w235:u32, "Error Out"=w237:errorcluster)  [unwired: 2 in, 14 out]
            n101 = call "Vision Research Phantom Series PhCon PhWriteStgFlash.vi"("CN in"=w235, "Error In (no error)"=w237) -> ("Error Out"=w236:errorcluster)  [unwired: 2 in, 15 out]
          }
        }
      }
      frame "CTS" {
        w256 = FALSE
        n102 = flat-sequence {
          tunnel: w249 -> [w280]
          tunnel: w246 -> [w281]
          tunnel: w247 -> [w282]
          tunnel: w248 -> [w283]
          tunnel: [w283] -> w244
          tunnel: [w282] -> w243
          tunnel: [w281] -> w242
          tunnel: [w280] -> w241
          tunnel: [w265] -> w240
          tunnel: [w290] -> w255
          tunnel: [w285] -> w254
          tunnel: [w288] -> w253
          tunnel: [w287] -> w252
          tunnel: w244 -> [w300]
          tunnel: w243 -> [w299]
          tunnel: w242 -> [w301]
          tunnel: w241 -> [w289]
          tunnel: w240 -> [w284]
          tunnel: w255 -> [w317]
          tunnel: w254 -> [w319]
          tunnel: w253 -> [w318]
          tunnel: [w316] -> w251
          tunnel: [w315] -> w250
          tunnel: w252 -> [_]
          tunnel: w251 -> [w322]
          tunnel: w250 -> [w323]
          tunnel: [w321] -> w245
          frame #0 {
            n103 = local read "Data run info"() -> (w264:T1)
            n104 = local read "Datarun timed out"() -> (w263:bool)
            n105 = Unbundle By Name(w264) -> ("Data run key"=w267:string, "Shot number"=w268:u32, "Timestamp"=w269:dbl)  [unwired: 1 out]
            n106 = Get Date/Time In Seconds() -> (seconds since 1Jan1904=w270:timestamp)
            n107 = Number To Decimal String(number=w268) -> (decimal integer string=w273:string)  [unwired: 1 in]
            n108 = Number To Decimal String(number=w269) -> (decimal integer string=w275:string)  [unwired: 1 in]
            n109 = Format Date/Time String(time format string (%c)="%Y-%m-%d-%H-%M-%S-%3u.cine", seconds (now)=w270) -> (date/time string=w277:string)  [unwired: 1 in]
            n110 = Concatenate Strings(w267, "-shot ", w273, "-time ", w275, ".cine") -> (w278:string)
            n111 = Select(t=w277, s=w263, f=w278) -> (s? t:f=w279:string)
            n112 = Build Path(base path=path "C:/Users/daq/Desktop/Saved Cines", name or relative path=w279) -> (appended path=w265:path)
            "Save path" <- w265
          }
          frame #1 {
            w295 = T18 506 items=["GCI_CFA"=0, "GCI_FRAMERATE"=1, "GCI_EXPOSURE"=2, "GCI_AUTOEXPOSURE"=3, "GCI_REALBPP"=4, "GCI_CAMERASERIAL"=5, "GCI_HEADSERIAL0"=6, "GCI_HEADSERIAL1"=7, "GCI_HEADSERIAL2"=8, "GCI_HEADSERIAL3"=9, "GCI_TRIGTIMESEC"=10, "GCI_TRIGTIMEFR"=11, "GCI_ISFILECINE"=12, "GCI_IS16BPPCINE"=13, "GCI_ISCOLORCINE"=14, "GCI_ISMULTIHEADCINE"=15, "GCI_EXPOSURENS"=16, "GCI_EDREXPOSURENS"=17, "GCI_FRAMEDELAYNS"=19, "GCI_FROMFILETYPE"=20, "GCI_COMPRESSION"=21, "GCI_CAMERAVERSION"=22, "GCI_ROTATE"=23, "GCI_IMWIDTH"=24, "GCI_IMHEIGHT"=25, "GCI_IMWIDTHACQ"=26, "GCI_IMHEIGHTACQ"=27, "GCI_POSTTRIGGER"=28, "GCI_IMAGECOUNT"=29, "GCI_TOTALIMAGECOUNT"=30, "GCI_TRIGFRAME"=31, "GCI_AUTOEXPLEVEL"=32, "GCI_AUTOEXPTOP"=33, "GCI_AUTOEXPLEFT"=34, "GCI_AUTOEXPBOTTOM"=35, "GCI_AUTOEXPRIGHT"=36, "GCI_RECORDINGTIMEZONE"=37, "GCI_FIRSTIMAGENO"=38, "GCI_FIRSTMOVIEIMAGE"=39, "GCI_CINENAME"=40, "GCI_FRPSTEPS"=100, "GCI_FRP1X"=101, "GCI_FRP1Y"=102, "GCI_FRP2X"=103, "GCI_FRP2Y"=104, "GCI_FRP3X"=105, "GCI_FRP3Y"=106, "GCI_FRP4X"=107, "GCI_FRP4Y"=108, "GCI_WRITEERR"=109, "GCI_LENSDESCRIPTION"=110, "GCI_LENSAPERATURE"=111, "GCI_LENSFOCALLENGTH"=112, "GCI_WB"=200, "GCI_WBVIEW"=201, "GCI_BRIGHT"=202, "GCI_CONTRAST"=203, "GCI_GAMMA"=204, "GCI_GAMMAR"=223, "GCI_GAMMAB"=224, "GCI_SATURATION"=205, "GCI_HUE"=206, "GCI_FLIPH"=207, "GCI_FLIPV"=208, "GCI_FILTERCODE"=209, "GCI_IMFILTER"=210, "GCI_INTALGO"=211, "GCI_PEDESTALR"=212, "GCI_PEDESTALG"=213, "GCI_PEDESTALB"=214, "GCI_FLARE"=225, "GCI_CHROMA"=226, "GCI_TONE"=227, "GCI_ENABLEMATRICES"=228, "GCI_USERMATRIX"=229, "GCI_RESAMPLEACTIVE"=215, "GCI_RESAMPLEWIDTH"=216, "GCI_RESAMPLEHEIGHT"=217, "GCI_CROPACTIVE"=218, "GCI_CROPRECTANGLE"=219, "GCI_OFFSET16_8"=220, "GCI_GAIN16_8"=221, "GCI_DEMOSAICINGFUNCPTR"=222, "GCI_VFLIPVIEWACTIVE"=300, "GCI_MAXIMGSIZE"=400, "GCI_FRPIMGNOARRAY"=450, "GCI_FRPRATEARRAY"=451, "GCI_FRPSHAPEARRAY"=452, "GCI_TRIGTC"=470, "GCI_TRIGTCU"=471, "GCI_PBRATE"=472, "GCI_TCRATE"=473, "GCI_SAVERANGE"=500, "GCI_SAVEFILENAME"=501, "GCI_SAVEFILETYPE"=502, "GCI_SAVE16BIT"=503, "GCI_SAVEPACKED"=504, "GCI_SAVEXML"=505, "GCI_SAVESTAMPTIME"=506, "GCI_SAVEAVIFRAMERATE"=520, "GCI_SAVEAVICOMPRESSORLIST"=521, "GCI_SAVEAVICOMPRESSORINDEX"=522, "GCI_SAVEDPXLSB"=530, "GCI_SAVEDPXTO10BPS"=531, "GCI_SAVEDPXDATAPACKING"=532, "GCI_SAVEDPX10BITLOG"=533, "GCI_SAVEDPXEXPORTLOGLUT"=534, "GCI_SAVEDPX10BITLOGREFWHITE"=535, "GCI_SAVEDPX10BITLOGREFBLACK"=536, "GCI_SAVEDPX10BITLOGGAMMA"=537, "GCI_SAVEDPX10BITLOGFILMGAMMA"=538, "GCI_SAVEQTPLAYBACKRATE"=550, "GCI_SAVECCIQUALITY"=560, "GCI_UNCALIBRATEDIMAGE"=600, "GCI_NOPROCESSING"=601, "GCI_BADPIXELREPAIR"=602] ("InfName [in]")
            n113 = call "Vision Research Phantom Series PhFile PhNewCineFromCamera.vi"("Camera Number in"=w301, "CineNr in"=1, "Error In (no error)"=w289) -> ("Camera Number out"=w288:u32, "CineNr out"=w285:i32, "pCH"=w286:u32, "Error Out"=w298:errorcluster)  [unwired: 2 in, 11 out]
            n114 = call "Vision Research Phantom Series PhFile PhSetCineSaveRange.vi"("CH in"=w286, "pFirstIm"=w300, "pLastIm"=w299, "Error In (no error)"=w298) -> ("CH out"=w297:u32, "Error Out"=w294:errorcluster)  [unwired: 14 in]
            n115 = call "Vision Research Phantom Series PhFile PhSetCineInfo.vi"("CH [in]"=w297, "InfName [in]"=w295, "pInfVal [in]"="Save StampTime", "Error In (no error)"=w294) -> ("CH [out]"=w293:u32, "Error Out"=w292:errorcluster)  [unwired: 1 in, 13 out]
            n116 = call "Vision Research Phantom Series PhFile PhSetCineSaveOptions.vi"("CH in"=w293, "szFileName"=w284, "Error In (no error)"=w292) -> ("CH out"=w287:u32, "Error Out"=w291:errorcluster)  [unwired: 15 in]
            n117 = case shown="No Error" w291 {
              tunnel: w291 -> [w305 w314]
              tunnel: w287 -> [w304 _]
              tunnel: [w303 w314] -> w290
              frame No Error {
                n118 = while {
                  tunnel: w305 -> [w311]
                  tunnel: w304 -> [w310]
                  stop <- w308 continue-if-true
                  n119 = call "Vision Research Phantom Series PhFile PhGetWriteCineFileProgress.vi"("CH [in]"=w310, "Error In (no error)"=w311) -> ("pProgressPercent [out]"=w307:u32, "Error Out"=w309:errorcluster)  [unwired: 1 in, 15 out]
                  n120 = Wait (ms)(milliseconds to wait=u32 100) -> ()  [unwired: 1 out]
                  n121 = local write "Save Progress"(w307) -> ()
                  n122 = case shown="Error" w309 {
                    tunnel: [TRUE FALSE] -> w308
                    frame No Error {
                    }
                    frame Error {
                    }
                  }
                }
                n123 = call "Vision Research Phantom Series PhFile PhWriteCineFile.vi"("CH in"=w304, "Error In (no error)"=w305) -> ("Error Out"=w303:errorcluster)  [unwired: 2 in, 15 out]
              }
              frame Error {
              }
            }
          }
          frame #2 {
            n124 = call "Vision Research Phantom Series PhCon PhDeleteCine.vi"("CN in"=w318, "Cine"=w319, "Error In (no error)"=w317) -> ("CN out"=w315:u32, "Error Out"=w316:errorcluster)  [unwired: 15 in]
          }
          frame #3 {
            n125 = call "Vision Research Phantom Series PhCon PhRecordCine.vi"("CN in"=w323, "Error In (no error)"=w322) -> ("Error Out"=w321:errorcluster)  [unwired: 16 in, 1 out]
            n126 = Wait (ms)(milliseconds to wait=u32 100) -> ()  [unwired: 1 out]
          }
        }
        n127 = local write "Recording"(w256) -> ()
        n128 = local write "Trigger"(w256) -> ()
        n129 = call "Vision Research Phantom Series PhCon PhDeleteCine.vi"("CN in"=u32 0, "Cine"=1 ("CineNr in"), "Error In (no error)"=w245) -> ("CN out"=w259:u32, "Error Out"=w260:errorcluster)  [unwired: 15 in]
        n130 = call "Vision Research Phantom Series PhCon PhRecordCine.vi"("CN in"=w259, "Error In (no error)"=w260) -> ("Error Out"=w262:errorcluster)  [unwired: 16 in, 1 out]
      }
      frame "Review" {
      }
      frame "End" {
        w328 = FALSE ("Continue")
        n131 = call "Vision Research Phantom Series Close.vi"("Error In (no error)"=w329) -> ("Error Out"=w327:errorcluster)  [unwired: 1 in, 17 out]
        n132 = local write "EXIT"(w328) -> ()
        n133 = property on="Preview" class="Pict"("ZoomFactor"=sgl 1.0 ("Zoom Factor")) -> ()  [unwired: 2 in, 2 out]
        "Continue" <- w328
      }
    }
    "state" <- w41
  }
  "Error" <- w13
